vi "Set Target Position.vi"(9 "Control Mode":T9 items=["PercentOutput"=0, "Position"=1, "Velocity"=2, "Current"=3, "Follower"=5, "MotionProfile"=6, "MotionMagic"=7, "MotionProfileArc"=10, "Disabled"=15], 10 "Input (deg)":cluster{"LF":dbl, "LB":dbl, "RF":dbl, "RB":dbl}, 11 "Swerve motors":cluster{"LF":T2, "LB":T2, "RF":T2, "RB":T2}) -> (3 "output cluster":T7)   [LabVIEW 2020]
uses:
  <vilib>/Rock Robotics/WPI/MotorControl/WPI_MotorControlDeviceRef.ctl
  <vilib>/Rock Robotics/WPI/MotorControl/WPI_MotorControlType.ctl
  <vilib>/Rock Robotics/SystemInterfaces/DIO/FPGA_DIOPWMChannel.ctl
  <vilib>/Rock Robotics/WPI/PWM/WPI_PWMDeadband.ctl
  <vilib>/Rock Robotics/SystemInterfaces/DIO/FPGA_DIOChannel.ctl
  <vilib>/Rock Robotics/WPI/ThirdParty/Phoenix-LabVIEW/Motor Controller/Controls/CTRE_Phoenix_MotorControl_ControlMode.ctl
  66f59f0f-3b86-4884-8eb4-07b41df825aa.vi
  <vilib>/Rock Robotics/WPI/ThirdParty/Phoenix-LabVIEW/Motor Controller/Get/CTRE_Phoenix_MotorController_GetSelectedSensorData.vi
  Framework/Robot Global Data.vi
panel:
  in  "Current Pod":T1(ring)
  in  "Push PID":bool
  out "Position\nErrors":T8(graph)
  in  "Debug Mode":bool
  in  "F":dbl
  in  "D":dbl
  in  "I":dbl
  in  "P":dbl
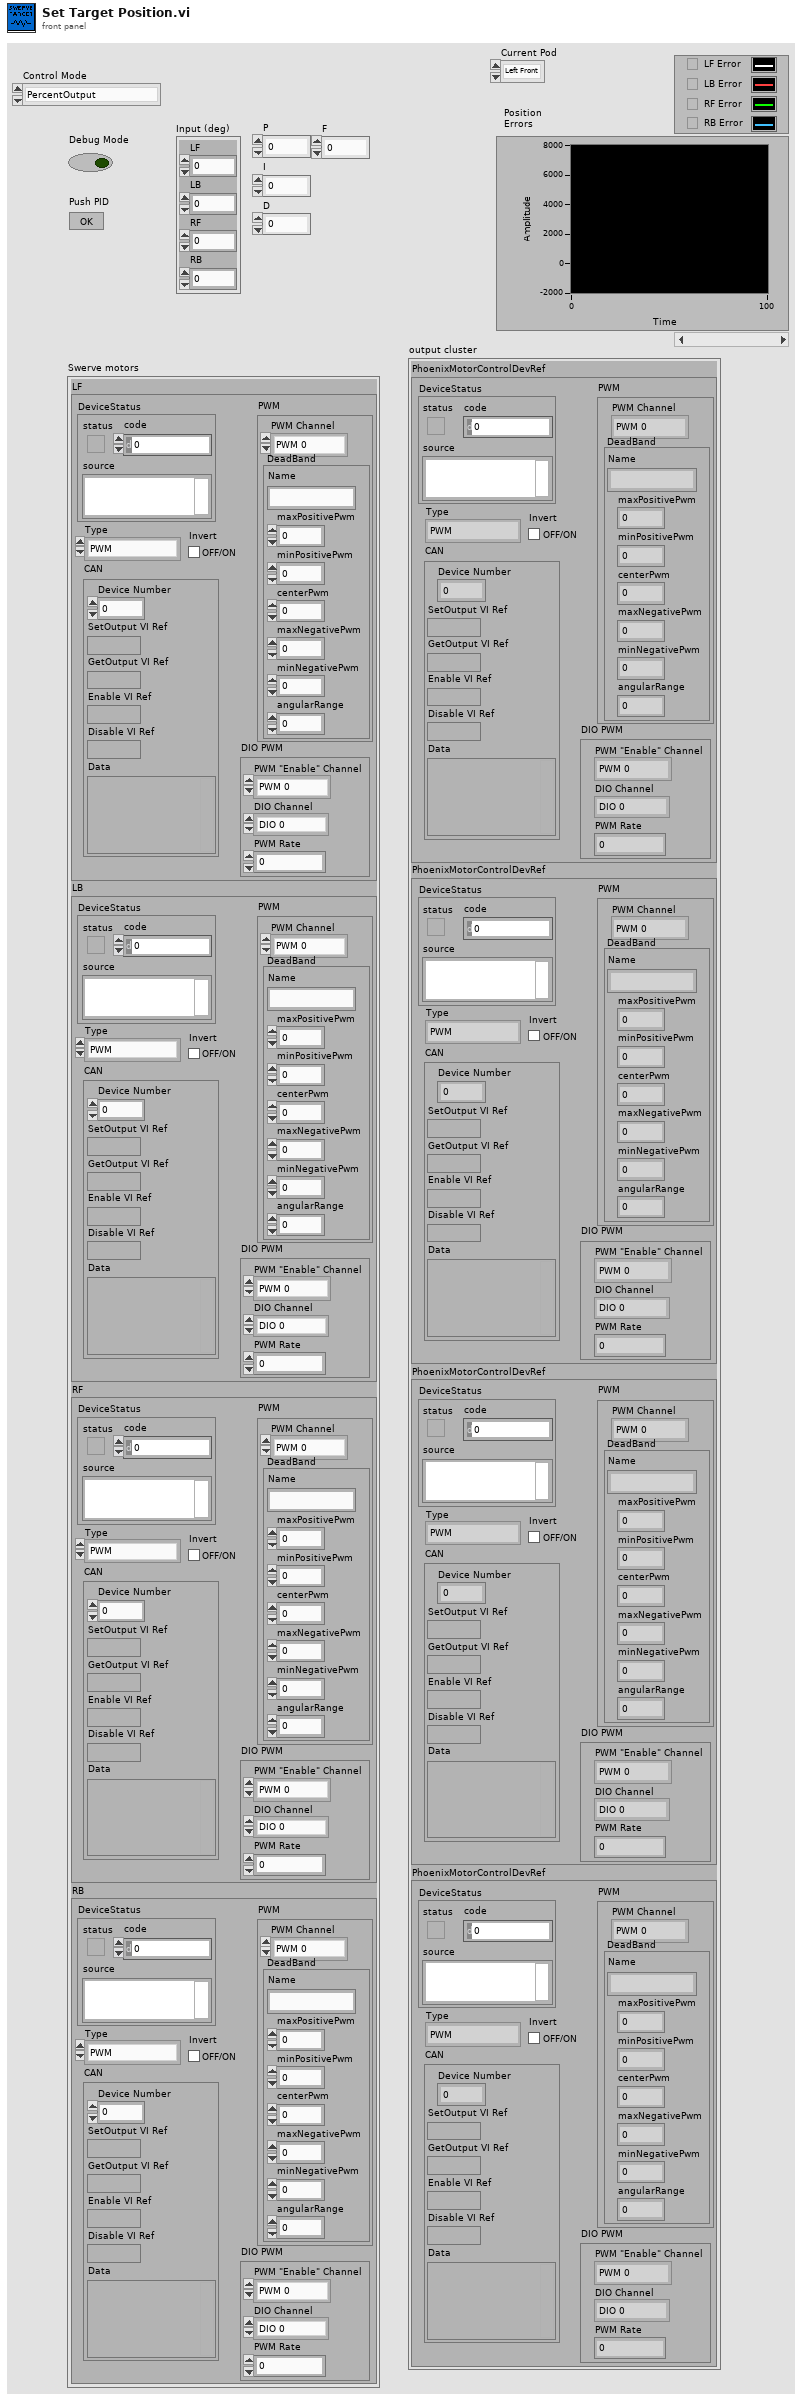
[diagram p1: front panel]
types:
  T1 = enum16{"Left Front", "Left Back", "Right Front", "Right Back"}
  T2 = typedef "WPI_MotorControlDeviceRef.ctl" = cluster{"DeviceStatus":errorcluster, "Type":T3, "PWM":cluster{"PWM Channel":T4, "DeadBand":T5}, "CAN":cluster{"Device Number":u8, "SetOutput VI Ref":variant, "GetOutput VI Ref":variant, "Enable VI Ref":variant, "Disable VI Ref":variant, "Data":variant}, "Invert":bool, "DIO PWM":cluster{"PWM \"Enable\" Channel":T4, "DIOChannel":T6, "PWM Rate":dbl}}
  T3 = typedef "WPI_MotorControlType.ctl" = enum16{"PWM", "CAN", "DIO PWM"}
  T4 = typedef "FPGA_DIOPWMChannel.ctl" = enum8{"PWM 0", "PWM 1", "PWM 2", "PWM 3", "PWM 4", "PWM 5", "PWM 6", "PWM 7", "PWM 8", "PWM 9", "PWM MXP 0", "PWM MXP 1", "PWM MXP 2", "PWM MXP 3", "PWM MXP 4", "PWM MXP 5", "PWM MXP 6", "PWM MXP 7", "PWM MXP 8", "PWM MXP 9", "Invalid"}
  T5 = typedef "WPI_PWMDeadband.ctl" = cluster{"Name":string, "maxPositivePwm":i32, "minPositivePwm":i32, "centerPwm":i32, "maxNegativePwm":i32, "minNegativePwm":i32, "angularRange":u16}
  T6 = typedef "FPGA_DIOChannel.ctl" = enum8{"DIO 0", "DIO 1", "DIO 2", "DIO 3", "DIO 4", "DIO 5", "DIO 6", "DIO 7", "DIO 8", "DIO 9", "DIO MXP 0", "DIO MXP 1", "DIO MXP 2", "DIO MXP 3", "DIO MXP 4", "DIO MXP 5", "DIO MXP 6", "DIO MXP 7", "DIO MXP 8", "DIO MXP 9", "DIO MXP 10", "DIO MXP 11", "DIO MXP 12", "DIO MXP 13", "DIO MXP 14", "DIO MXP 15", "SPI Port CS1", "SPI Port CS2", "SPI Port CS3", "SPI Port MISO", "SPI Port MOSI", "Invalid"}
  T7 = cluster{"PhoenixMotorControlDevRef":T2, "PhoenixMotorControlDevRef":T2, "PhoenixMotorControlDevRef":T2, "PhoenixMotorControlDevRef":T2}
  T8 = cluster{"Position (Raw Sensor Units)":i32, "ticks":dbl}
  T9 = typedef "CTRE_Phoenix_MotorControl_ControlMode.ctl" = u16
  T10 = cluster{"LF":bool, "LB":bool, "RF":bool, "RB":bool}
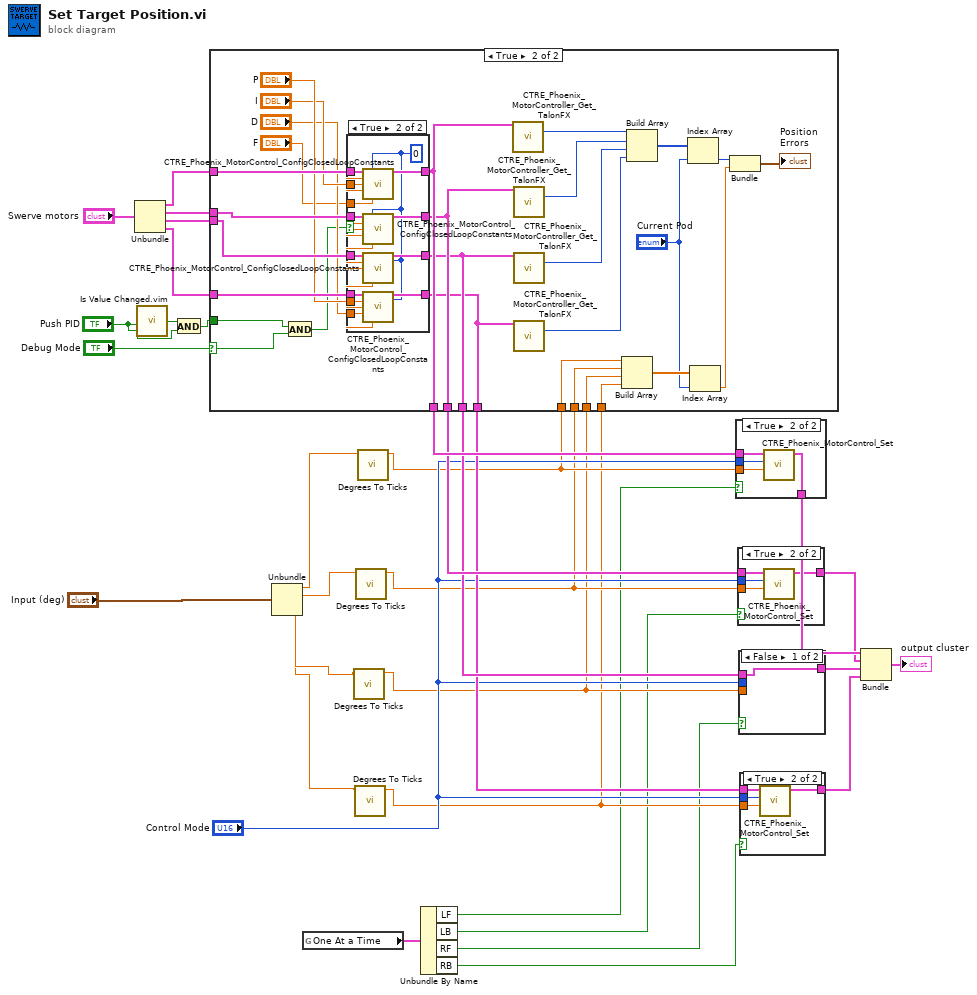
[diagram p0: block diagram]
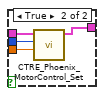
[diagram p3: hidden frame]
diagram:
  n1 = Unbundle("Swerve motors") -> ("LF"=w32:T2, "LB"=w31:T2, "RF"=w30:T2, "RB"=w29:T2)
  n2 = call "Is Value Changed.vim"("value"="Push PID") -> ("changed or first call?"=w22:bool)
  n3 = And(x=w22, y="Push PID") -> (x .and. y?=w20:bool)
  n4 = Unbundle("Input (deg)") -> ("LF"=w19:dbl, "LB"=w17:dbl, "RF"=w15:dbl, "RB"=w13:dbl)
  n5 = global read "Robot Global Data.vi" "One At a Time"() -> (w6:T10)
  n6 = call "Degrees To Ticks.vi"("degrees"=w15) -> ("ticks"=w14:dbl)  [unwired: 10 in]
  n7 = call "Degrees To Ticks.vi"("degrees"=w13) -> ("ticks"=w12:dbl)  [unwired: 10 in]
  n8 = call "Degrees To Ticks.vi"("degrees"=w17) -> ("ticks"=w16:dbl)  [unwired: 10 in]
  n9 = call "Degrees To Ticks.vi"("degrees"=w19) -> ("ticks"=w18:dbl)  [unwired: 10 in]
  n10 = case shown="True" "Debug Mode" {
    selector: "Debug Mode" -> [_ w52]
    tunnel: w32 -> [w37 w66]
    tunnel: w31 -> [w36 w65]
    tunnel: w30 -> [w35 w64]
    tunnel: w29 -> [w34 w63]
    tunnel: [w37 w58] -> w28
    tunnel: [w36 w57] -> w27
    tunnel: [w35 w56] -> w26
    tunnel: [w34 w55] -> w25
    tunnel: w18 -> [_ w39]
    tunnel: w16 -> [_ w40]
    tunnel: w14 -> [_ w41]
    tunnel: w12 -> [_ w42]
    tunnel: w20 -> [_ w53]
    frame False {
    }
    frame True {
      n11 = And(x=w53, y=w52) -> (x .and. y?=w54:bool)
      n12 = case shown="True" w54 {
        tunnel: w66 -> [w70 w83]
        tunnel: w65 -> [w69 w82]
        tunnel: w64 -> [w68 w81]
        tunnel: w63 -> [w67 w80]
        tunnel: "P" -> [_ w79]
        tunnel: "I" -> [_ w78]
        tunnel: "D" -> [_ w77]
        tunnel: "F" -> [_ w76]
        tunnel: [w70 w75] -> w58
        tunnel: [w69 w74] -> w57
        tunnel: [w68 w73] -> w56
        tunnel: [w67 w72] -> w55
        frame False {
        }
        frame True {
          w71 = 0 ("slotIdx")
          n13 = call <vilib>:"CTRE_Phoenix_MotorControl_ConfigClosedLoopConstants.vi"("PhoenixMotorControlDevRef"=w83, "slotIdx"=w71, "P"=w79, "I"=w78, "D"=w77, "F"=w76) -> ("PhoenixMotorControlDevRef"=w75:T2)  [unwired: 8 in, 1 out]
          n14 = call <vilib>:"CTRE_Phoenix_MotorControl_ConfigClosedLoopConstants.vi"("PhoenixMotorControlDevRef"=w82, "slotIdx"=w71, "P"=w79, "I"=w78, "D"=w77, "F"=w76) -> ("PhoenixMotorControlDevRef"=w74:T2)  [unwired: 8 in, 1 out]
          n15 = call <vilib>:"CTRE_Phoenix_MotorControl_ConfigClosedLoopConstants.vi"("PhoenixMotorControlDevRef"=w81, "slotIdx"=w71, "P"=w79, "I"=w78, "F"=w76) -> ("PhoenixMotorControlDevRef"=w73:T2)  [unwired: 9 in, 1 out]
          n16 = call <vilib>:"CTRE_Phoenix_MotorControl_ConfigClosedLoopConstants.vi"("PhoenixMotorControlDevRef"=w80, "slotIdx"=w71, "P"=w79, "I"=w78, "D"=w77, "F"=w76) -> ("PhoenixMotorControlDevRef"=w72:T2)  [unwired: 8 in, 1 out]
        }
      }
      n17 = call-poly <vilib>:"CTRE_Phoenix_MotorController_Get_TalonFX.vi"("PhoenixMotorControlDevRef"=w58) -> ("Position (Raw Sensor Units)"=w46:i32)  [unwired: 11 in, 3 out]
      n18 = call-poly <vilib>:"CTRE_Phoenix_MotorController_Get_TalonFX.vi"("PhoenixMotorControlDevRef"=w57) -> ("Position (Raw Sensor Units)"=w45:i32)  [unwired: 11 in, 3 out]
      n19 = call-poly <vilib>:"CTRE_Phoenix_MotorController_Get_TalonFX.vi"("PhoenixMotorControlDevRef"=w56) -> ("Position (Raw Sensor Units)"=w44:i32)  [unwired: 11 in, 3 out]
      n20 = call-poly <vilib>:"CTRE_Phoenix_MotorController_Get_TalonFX.vi"("PhoenixMotorControlDevRef"=w55) -> ("Position (Raw Sensor Units)"=w43:i32)  [unwired: 11 in, 3 out]
      n21 = Build Array(w39, w40, w41, w42) -> (w50:dbl[])
      n22 = Build Array(w46, w45, w44, w43) -> (w51:i32[])
      n23 = Index Array(array=w51, index="Current Pod") -> (element=w49:i32)
      n24 = Index Array(array=w50, index="Current Pod") -> (element=w48:dbl)
      n25 = Bundle("Position (Raw Sensor Units)"=w49, "ticks"=w48) -> (→"Position\nErrors":T8)  [unwired: 1 in]
    }
  }
  n26 = Unbundle By Name(w6) -> ("LF"=w5:bool, "LB"=w4:bool, "RF"=w3:bool, "RB"=w2:bool)
  n27 = case shown="True" w5 {
    tunnel: w28 -> [w84 w88]
    tunnel: "Control Mode" -> [_ w87]
    tunnel: w18 -> [_ w86]
    tunnel: [w84 w85] -> w11
    frame False {
    }
    frame True {
      n28 = call <vilib>:"CTRE_Phoenix_MotorControl_Set.vi"("Output"=w86, "Control Mode"=w87, "PhoenixMotorControlDevRef"=w88) -> ("PhoenixMotorControlDevRef"=w85:T2)  [unwired: 7 in, 1 out]
    }
  }
  n29 = case shown="True" w4 {
    tunnel: w27 -> [w89 w93]
    tunnel: "Control Mode" -> [_ w92]
    tunnel: w16 -> [_ w91]
    tunnel: [w89 w90] -> w10
    frame False {
    }
    frame True {
      n30 = call <vilib>:"CTRE_Phoenix_MotorControl_Set.vi"("Output"=w91, "Control Mode"=w92, "PhoenixMotorControlDevRef"=w93) -> ("PhoenixMotorControlDevRef"=w90:T2)  [unwired: 7 in, 1 out]
    }
  }
  n31 = case shown="False" w3 {
    tunnel: w26 -> [w94 w98]
    tunnel: "Control Mode" -> [_ w97]
    tunnel: w14 -> [_ w96]
    tunnel: [w94 w95] -> w9
    frame False {
    }
    frame True {
      n32 = call <vilib>:"CTRE_Phoenix_MotorControl_Set.vi"("Output"=w96, "Control Mode"=w97, "PhoenixMotorControlDevRef"=w98) -> ("PhoenixMotorControlDevRef"=w95:T2)  [unwired: 7 in, 1 out]
    }
  }
  n33 = case shown="True" w2 {
    tunnel: w25 -> [w99 w103]
    tunnel: "Control Mode" -> [_ w102]
    tunnel: w12 -> [_ w101]
    tunnel: [w99 w100] -> w8
    frame False {
    }
    frame True {
      n34 = call <vilib>:"CTRE_Phoenix_MotorControl_Set.vi"("Output"=w101, "Control Mode"=w102, "PhoenixMotorControlDevRef"=w103) -> ("PhoenixMotorControlDevRef"=w100:T2)  [unwired: 7 in, 1 out]
    }
  }
  n35 = Bundle("PhoenixMotorControlDevRef"=w11, "PhoenixMotorControlDevRef"=w10, "PhoenixMotorControlDevRef"=w9, "PhoenixMotorControlDevRef"=w8) -> (→"output cluster":T7)  [unwired: 1 in]
